vi "WriteGraphSettings.vi"(8 "Error In":errorcluster, 10 "Value":string, 11 "Key":string) -> (0 "Error Out":errorcluster)   [LabVIEW 2018]
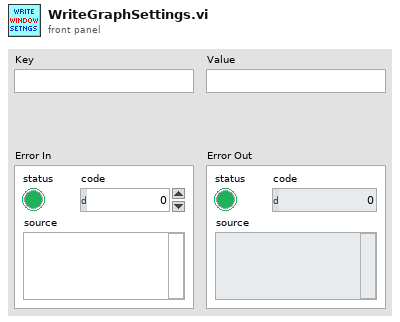
[diagram p1: front panel]
types:
  T1 = enum16{"open", "replace", "create", "open or create", "replace or create", "replace or create with confirmation"}
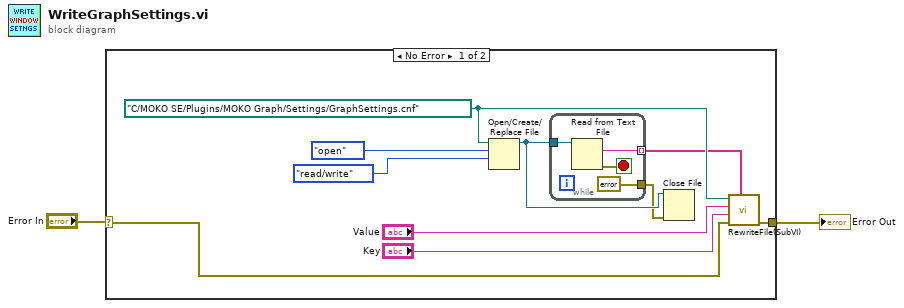
[diagram p0: block diagram]
diagram:
  n1 = case shown="No Error" "Error In" {
    selector: "Error In" -> [w5 w17]
    tunnel: [w4 w17] -> w1
    frame No Error {
      w7 = path "C:/MOKO SE/Plugins/MOKO Graph/Settings/GraphSettings.cnf" ("file path (use dialog)")
      n2 = Open/Create/Replace File(file path (use dialog)=w7, operation (0:open)=T1."open", access (0:read/write)=enum16{"read/write", "read-only", "write-only"}."read/write") -> (refnum out=w8:refnum<file>)  [unwired: 3 in, 2 out]
      n3 = while {
        tunnel: w8 -> [w16]
        tunnel: [w15] -> w6 mode=indexing
        tunnel: [errorcluster {"status"=FALSE, "code"=0, "source"=""} ("error out")] -> w3
        stop <- w14 stop-if-true
        n4 = Read from Text File(file (use dialog)=w16) -> (text=w15:string, error out=w14:errorcluster)  [unwired: 3 in, 2 out]
      }
      n5 = Close File(refnum=w8, error in=w3) -> ()  [unwired: 2 out]
      n6 = call "RewriteFile(SubVI).vi"("Content from file"=w6, "Error In"=w5, "Key"="Key", "Value"="Value", "file path (use dialog)"=w7) -> ("Error Out"=w4:errorcluster)  [unwired: 6 in]
    }
    frame Error {
    }
  }
  "Error Out" <- w1
